vi "FSK_main.vi"() -> ()   [LabVIEW 2015]
uses:
  LabviewSubVI/RFConfig/RF_Config.ctl
  LabviewSubVI/RFConfig/StudentMsg.ctl
panel:
  in  "载波2频率":dbl(ring)=2048.0 items=["4096Hz"=4096.0, "2048Hz"=2048.0]
  in  "载波1频率":dbl(ring)=512.0 items=["1024Hz"=1024.0, "512Hz"=512.0]
  out "FSK接收信号频谱":cluster{"w":dbl[], "SendSig_F":dbl[]}(graph)
  out "当前帧号":i32
  out "总误码数（每帧卷积译码后误码数累加）":dbl
  out "总误码率(每帧卷积译码后误码率的平均值)":dbl
  in  "信道类型":enum16{"理想信道", "非理想信道"}(ring)
  out "当前帧卷积译码后误码率":dbl
  out "当前帧卷积译码后误码数":dbl
  out "信宿":dbl[](array[numeric]) format="%#_13g"
  out "实验学生信息":T1={"姓名"="XXX\n", "学号"="XXX", "班级"="XXX", "学校"="XXX"}
  in  "运行方式":enum16{"仿真系统", "真实系统"}(ring)
  in  "?":T2={"发射频率"=2380000000, "发射衰减"=30, "接收频率"=2380000000, "接收增益"=12, "接收通道"=enum."RxCh1", "发射通道"=enum."TxCh1"} {"接收增益" max=40 format="%.0fdB"; "接收频率" min=70000000 max=6000000000 format="%.6pHz"; "发射衰减" max=90 format="%.0fdB"; "发射频率" min=70000000 max=6000000000 format="%.6pHz"}
  in  "XSRP IP":string="192.168.1.166"
  in  "运行次数":u8=1 min=1 max=100 step=1
  out "信源比特":dbl[](array[numeric]) format="%#_13g"
  out "FSK发送信号波形":dbl[](graph)
  out "FSK发送信号频谱":cluster{"w":dbl[], "SendSig_F":dbl[]}(graph)
  out "FSK接收信号波形":dbl[](graph)
  out "搜索同步码结果":dbl[][](graph)
  out "当前帧卷积译码前误码率":dbl
  out "当前帧卷积译码前误码数":dbl
  in  "非理性\n信道参数":T3={" 增益"=1.0, " 时延(s)"=0.0, " 频偏(Hz)"=0.0, " 相移(rad)"=0.0, " 信噪比(dB)"=40.0} {"信噪比(dB)" min=-20.0 max=40.0 step=1.0 format="%#_13g"; "相移(rad)" min=0.0 max=6.28 step=0.001 format="%#_13g"; "频偏(Hz)" min=0.0 max=100.0 step=1.0 format="%#_13g"; "时延(s)" min=0.0 max=0.2 step=0.001 format="%#_13g"; "增益" min=0.5 max=1.5 step=0.1 format="%#_13g"}
  in  "PC IP":string="192.168.1.180"
  # "基于XSRP软件无线电平台的FSK数字调制通信系统"
  # "实验参数设置"
  # "实验学生信息"
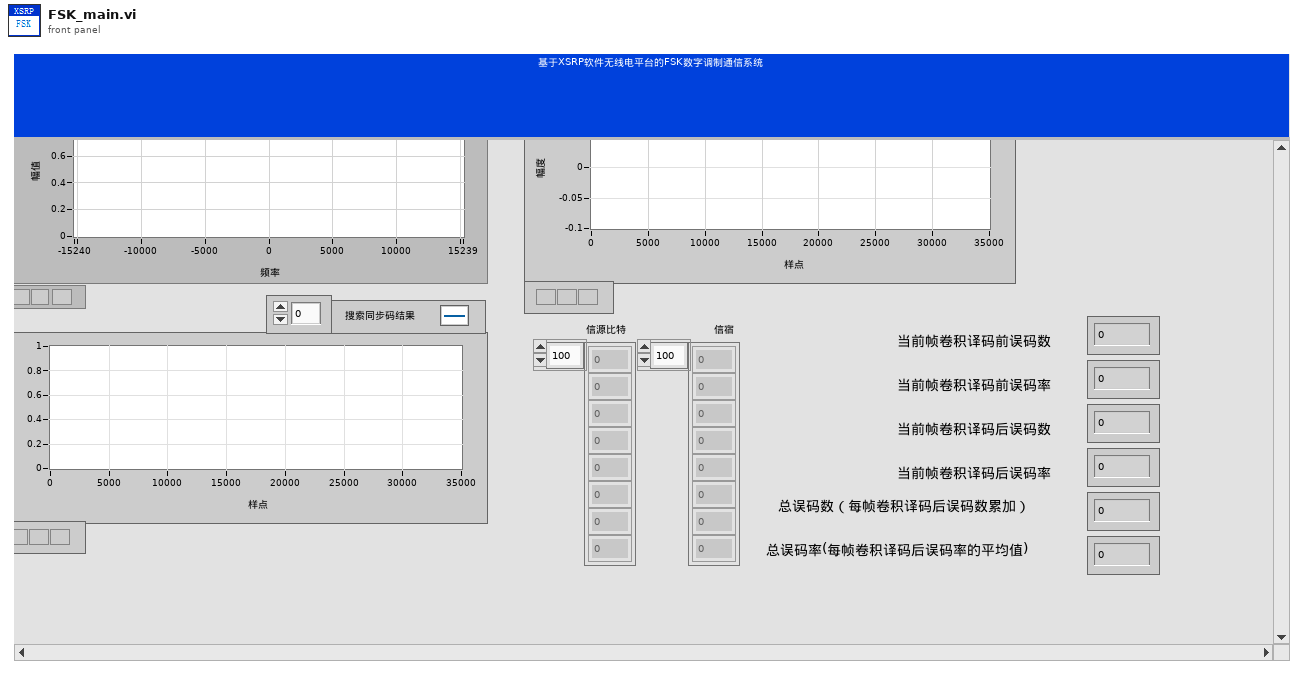
[diagram p1: front panel]
types:
  T1 = typedef "StudentMsg.ctl" = cluster{"姓名":string, "学号":string, "班级":string, "学校":string}
  T2 = typedef "RF_Config.ctl" = cluster{"发射频率":u64, "发射衰减":u8, "接收频率":u64, "接收增益":u8, "接收通道":enum16{"RxCh1", "RxCh2"}, "发射通道":enum16{"TxCh1", "TxCh2"}}
  T3 = cluster{" 增益":dbl, " 时延(s)":dbl, " 频偏(Hz)":dbl, " 相移(rad)":dbl, " 信噪比(dB)":dbl}
  T4 = cluster{"接收通道":enum16{"RxCh1", "RxCh2"}, "接收频率":u32, "接收增益":u8}
  T5 = cluster{"发射通道":enum16{"TxCh1", "TxCh2"}, "发射频率":u32, "发射衰减":u8}
  T6 = enum8{"Enabled", "Disabled", "Disabled and Grayed Out"}
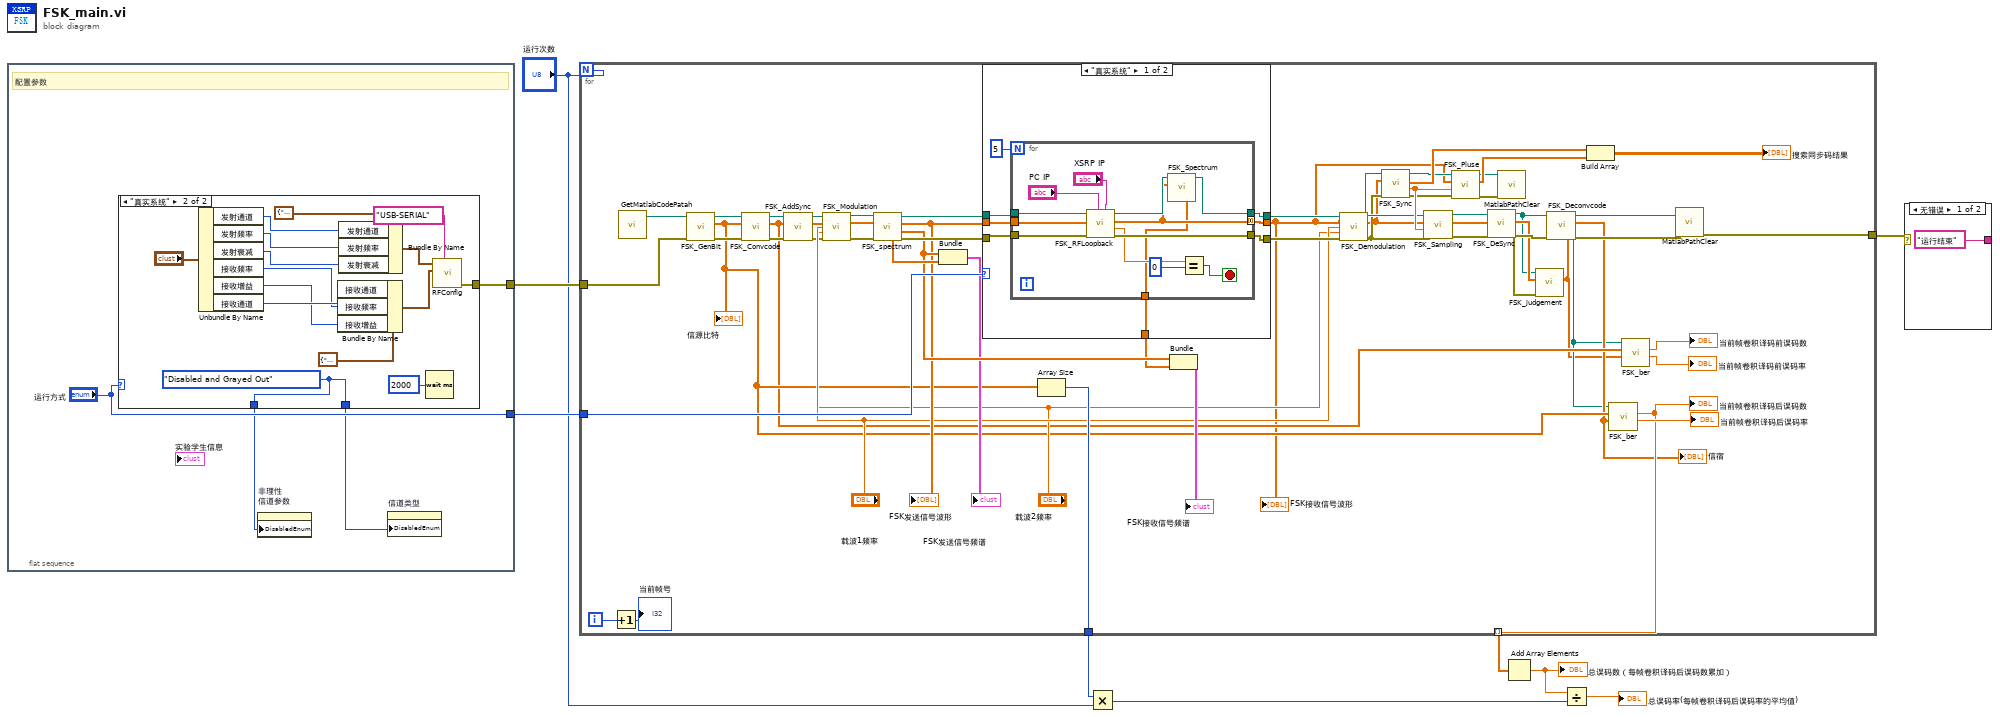
[diagram p0: block diagram]
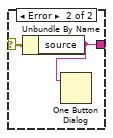
[diagram p2: hidden frame]
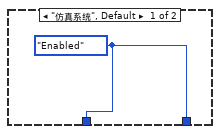
[diagram p3: hidden frame]
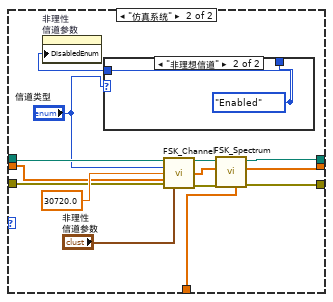
[diagram p4: hidden frame]
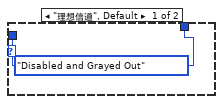
[diagram p5: hidden frame]
diagram:
  n1 = flat-sequence {
    tunnel: [w13] -> w9
    tunnel: ["运行方式"] -> w8
    frame #0 {
      # "配置参数"
      n2 = case shown="\"真实系统\"" "运行方式" {
        tunnel: [_ w18] -> w13
        tunnel: [w14 w15] -> w10
        tunnel: [w14 w15] -> w11
        frame "仿真系统", Default {
          w14 = T6."Enabled" ("Disabled")
        }
        frame "真实系统" {
          w15 = T6."Disabled and Grayed Out" ("Disabled")
          n3 = Unbundle By Name("?") -> ("发射通道"=w26:enum16{"TxCh1", "TxCh2"}, "发射频率"=w25:u64, "发射衰减"=w24:u8, "接收频率"=w20:u64, "接收增益"=w21:u8, "接收通道"=w22:enum16{"RxCh1", "RxCh2"})
          n4 = Bundle By Name(cluster=T4 {"接收通道"=enum."RxCh1", "接收频率"=0, "接收增益"=0} ("接收参数设置"), "接收通道"=w22, "接收频率"=w20, "接收增益"=w21) -> (w19:T4)
          n5 = Bundle By Name(cluster=T5 {"发射通道"=enum."TxCh1", "发射频率"=0, "发射衰减"=0} ("发射参数设置"), "发射通道"=w26, "发射频率"=w25, "发射衰减"=w24) -> (w28:T5)
          n6 = Wait (ms)(milliseconds to wait=u32 2000) -> ()  [unwired: 1 out]
          n7 = call "RFConfig.vi"("USB-SERIAL name"="USB-SERIAL", "接收参数设置"=w19, "发射参数设置"=w28) -> ("error out"=w18:errorcluster)  [unwired: 8 in]
        }
      }
      n8 = property on="非理性\n信道参数" class="Clust (严格)"("DisabledEnum"=w11) -> ()  [unwired: 2 in, 2 out]
      n9 = property on="信道类型" class="Enum (严格)"("DisabledEnum"=w10) -> ()  [unwired: 2 in, 2 out]
    }
  }
  n10 = for {
    N: "运行次数" -> [_]
    tunnel: w9 -> [w86]
    tunnel: w8 -> [w85]
    tunnel: [w82] -> w7
    tunnel: [w81] -> w5 mode=indexing
    tunnel: [w31] -> w1
    i -> [w80]
    n11 = Increment(x=w80) -> (x+1=→"当前帧号":i32)
    n12 = call "GetMatlabCodePatah.vi"() -> ("MatlabCodePath"=w78:path)  [unwired: 11 in]
    n13 = call "FSK_GenBit.vi"("error in (no error)"=w86, "PathIn"=w78) -> ("error out"=w76:errorcluster, "SendBit"=w49:dbl[], "PathOut"=w77:path)  [unwired: 7 in]
    "信源比特" <- w49
    n14 = call "FSK_Convcode.vi"("error in (no error)"=w76, "input_data"=w49, "PathIn"=w77) -> ("error out"=w58:errorcluster, "output_data"=w47:dbl[], "PathOut"=w60:path)  [unwired: 6 in]
    n15 = call "FSK_AddSync.vi"("error in (no error)"=w58, "code"=w47, "PathIn"=w60) -> ("error out"=w57:errorcluster, "data"=w56:dbl[], "PathOut"=w59:path)  [unwired: 6 in]
    n16 = call "FSK_Modulation.vi"("PathIn"=w59, "data"=w56, "FreqCarrier1"="载波1频率", "FreqCarrier2"="载波2频率", "error in (no error)"=w57) -> ("PathOut"=w75:path, "SendSig"=w74:cdb[], "error out"=w73:errorcluster)  [unwired: 8 in]
    n17 = call "FSK_spectrum.vi"("error in (no error)"=w73, "input_data"=w74, "PathIn"=w75) -> ("error out"=w71:errorcluster, "w"=w67:dbl[], "output_data"=w63:cdb[], "PathOut"=w72:path, "SendSig_F"=w70:dbl[])  [unwired: 4 in]
    "FSK发送信号波形" <- w63
    n18 = Bundle("w"=w67, "SendSig_F"=w70) -> (→"FSK发送信号频谱":cluster{"w":dbl[], "SendSig_F":dbl[]})  [unwired: 1 in]
    n19 = case shown="\"真实系统\"" w85 {
      tunnel: w63 -> [w94 w119]
      tunnel: w71 -> [w89 w118]
      tunnel: [w91 w108] -> w30
      tunnel: [w92 w113] -> w69
      tunnel: [w90 w109] -> w68
      tunnel: w72 -> [w93 w117]
      tunnel: [w87 w110] -> w65
      frame "真实系统" {
        n20 = for {
          N: 5 -> [_]
          tunnel: w94 -> [w99]
          tunnel: [w96] -> w91 mode=concatenating
          tunnel: w93 -> [w106]
          tunnel: [w97] -> w92
          tunnel: w89 -> [w103]
          tunnel: [w104] -> w90
          tunnel: [w95] -> w87
          stop <- w100 stop-if-true
          n21 = call "FSK_RFLoopback.vi"("xsrpip"="XSRP IP", "pcip"="PC IP", "error in (no error)"=w103, "SendSig"=w99, "PathIn"=w106) -> ("error out"=w104:errorcluster, "ERR_CODE"=w102:dbl, "RecvSig"=w96:cdb[], "PathOut"=w98:path)  [unwired: 3 in]
          n22 = call "FSK_Spectrum.vi"("input_data"=w96, "PathIn"=w98) -> ("PathOut"=w97:path, "SendSig_F"=w95:dbl[])  [unwired: 5 in, 3 out]
          n23 = Equal?(x=w102, y=0) -> (x = y?=w100:bool)
        }
      }
      frame "仿真系统" {
        n24 = case shown="\"非理想信道\"" "信道类型" {
          tunnel: [w122 w123] -> w115
          tunnel: [w122 w123] -> _
          frame "理想信道", Default {
            w122 = T6."Disabled and Grayed Out" ("Disabled")
          }
          frame "非理想信道" {
            w123 = T6."Enabled" ("Disabled")
          }
        }
        n25 = property on="非理性\n信道参数" class="Clust (严格)"("DisabledEnum"=w115) -> ()  [unwired: 2 in, 2 out]
        n26 = call "FSK_Channel.vi"("PathIn"=w117, "channel_flag"="信道类型", "Fs"=30720.0, "SendSig"=w119, "error in (no error)"=w118, "簇"="非理性\n信道参数") -> ("PathOut"=w114:path, "RecvSig"=w112:cdb[], "error out"=w111:errorcluster)  [unwired: 7 in]
        n27 = call "FSK_Spectrum.vi"("error in (no error)"=w111, "input_data"=w112, "PathIn"=w114) -> ("error out"=w109:errorcluster, "output_data"=w108:cdb[], "PathOut"=w113:path, "SendSig_F"=w110:dbl[])  [unwired: 4 in, 1 out]
      }
    }
    "FSK接收信号波形" <- w30
    n28 = Array Size(array=w49) -> (size(s)=w82:i32)
    n29 = Bundle("w"=w67, "SendSig_F"=w65) -> (→"FSK接收信号频谱":cluster{"w":dbl[], "SendSig_F":dbl[]})  [unwired: 1 in]
    n30 = call "FSK_Demodulation.vi"("PathIn"=w69, "input_data"=w30, "FreqCarrier1"="载波1频率", "FreqCarrier2"="载波2频率", "error in (no error)"=w68) -> ("PathOut"=w38:path, "RecvFskDemod"=w35:cdb[], "error out"=w37:errorcluster)  [unwired: 8 in]
    n31 = call "FSK_Sync.vi"("error in (no error)"=w37, "RecvFskDemod"=w35, "PathIn"=w38) -> ("error out"=w36:errorcluster, "pos"=w46:dbl, "RecvCorr"=w55:dbl[], "PathOut"=w54:path)  [unwired: 5 in]
    n32 = call "FSK_Sampling.vi"("error in (no error)"=w37, "pos"=w46, "RecvFskDemod"=w35, "PathIn"=w38) -> ("error out"=w45:errorcluster, "RecvSymbolSampled"=w43:dbl[], "PathOut"=w44:path)  [unwired: 5 in]
    n33 = call "FSK_Pluse.vi"("error in (no error)"=w36, "pos"=w46, "RecvSig"=w30, "PathIn"=w54) -> ("error out"=w33:errorcluster, "samplePulse"=w53:dbl[], "PathOut"=w34:path)  [unwired: 5 in]
    n34 = call "FSK_DeSync.vi"("error in (no error)"=w45, "RecvSymbolSampled"=w43, "PathIn"=w44) -> ("error out"=w52:errorcluster, "RecvDeSync"=w51:dbl[], "PathOut"=w50:path)  [unwired: 6 in]
    n35 = call "MatlabPathClear.vi"("error in"=w33, "Path"=w34) -> ()  [unwired: 9 in, 1 out]
    n36 = call "FSK_judgement.vi"("error in (no error)"=w52, "RecvDeSync"=w51, "PathIn"=w50) -> ("judgeSampled_data"=w32:dbl[])  [unwired: 6 in, 2 out]
    n37 = call "FSK_Deconvcode.vi"("error in (no error)"=w52, "RecvDeSync"=w32, "PathIn"=w50) -> ("error out"=w48:errorcluster, "RecvBit"=w42:dbl[], "PathOut"=w39:path)  [unwired: 6 in]
    "信宿" <- w42
    n38 = Build Array(w55, w53) -> (→"搜索同步码结果":dbl[][])
    n39 = call "FSK_ber.vi"("rxbit"=w42, "txbit"=w49, "Path In"=w39) -> ("ber"=→"当前帧卷积译码后误码率":dbl, "errnum"=w81:dbl)  [unwired: 5 in, 2 out]
    "当前帧卷积译码后误码数" <- w81
    n40 = call "FSK_ber.vi"("rxbit"=w32, "txbit"=w47, "Path In"=w39) -> ("ber"=→"当前帧卷积译码前误码率":dbl, "errnum"=→"当前帧卷积译码前误码数":dbl)  [unwired: 5 in, 2 out]
    n41 = call "MatlabPathClear.vi"("error in"=w48, "Path"=w39) -> ("error out"=w31:errorcluster)  [unwired: 9 in]
  }
  n42 = Multiply(x=w7, y="运行次数") -> (x*y=w3:i32)
  n43 = Add Array Elements(numeric array=w5) -> (sum=w4:dbl)
  "总误码数（每帧卷积译码后误码数累加）" <- w4
  n44 = Divide(x=w4, y=w3) -> (x/y=→"总误码率(每帧卷积译码后误码率的平均值)":dbl)
  n45 = case shown="无错误" w1 {
    selector: w1 -> [_ w126]
    tunnel: ["运行结束" ("source") w125] -> _
    frame No Error {
    }
    frame Error {
      n46 = Unbundle By Name(w126) -> ("source"=w125:string)
      n47 = One Button Dialog(message=w125) -> ()  [unwired: 1 in, 1 out]
    }
  }
